vi "Add Procedure.vi"(7 "Overwrite Existing?":bool=TRUE, 8 "error in (no error)":errorcluster, 9 "Settings":cluster{"Name":string}, 10 "Base Node Path":string, 11 "SysDef Ref":T1) -> (0 "error out":errorcluster, 2 "New Node Path":string, 3 "SysDef Ref Out":T1)   [LabVIEW 2019, in "Simple SysDef API.lvlib"]
uses:
  <userlib>/SimpleSysDef/Simple SysDef API.lvlib
  <userlib>/SimpleSysDef/_SubVIs/System Definition Reference.ctl
  NationalInstruments.VeriStand.SystemDefinitionAPI
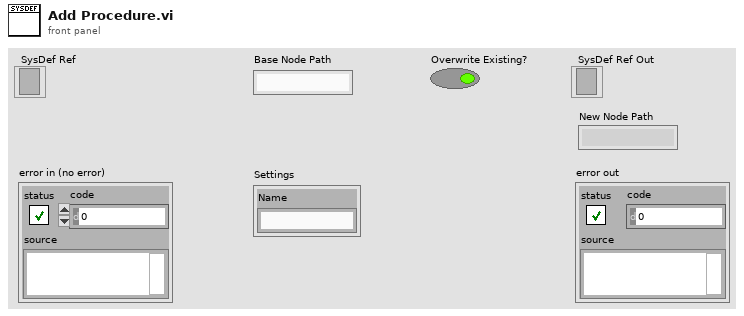
[diagram p1: front panel]
types:
  T1 = typedef "Simple SysDef API.lvlib/System Definition Reference.ctl" = refnum<k24>
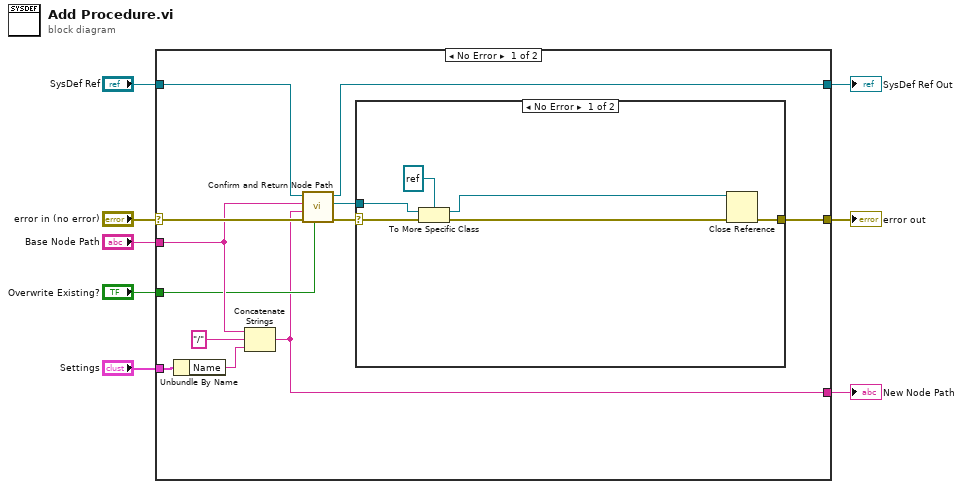
[diagram p0: block diagram]
diagram:
  n1 = case shown="No Error" "error in (no error)" {
    selector: "error in (no error)" -> [w20 w29]
    tunnel: [w14 w29] -> w7
    tunnel: "SysDef Ref" -> [w19 w28]
    tunnel: [w18 w28] -> w5
    tunnel: "Base Node Path" -> [w11 _]
    tunnel: "Overwrite Existing?" -> [w10 _]
    tunnel: "Settings" -> [w17 _]
    tunnel: [w9 _] -> w1
    frame No Error {
      n2 = Unbundle By Name(w17) -> ("Name"=w15:string)
      n3 = Concatenate Strings(w11, "/" ("string"), w15) -> (w9:string)
      n4 = call <userlib>:"Confirm and Return Node Path.vi"("Overwrite Existing?"=w10, "error in (no error)"=w20, "New Node Path"=w9, "Base Node Path"=w11, "SysDef Ref"=w19) -> ("error out"=w12:errorcluster, "Node Ref"=w13:refnum<k24>, "SysDef Ref Out"=w18:T1)  [unwired: 4 in]
      n5 = case shown="No Error" w12 {
        selector: w12 -> [w25 w27]
        tunnel: [w23 w27] -> w14
        tunnel: w13 -> [w26 _]
        frame No Error {
          n6 = To More Specific Class(target class=refnum<k24> refnum ("Node Ref"), reference=w26, error in=w25) -> (specific class reference=w22:refnum<k24>, error out=w24:errorcluster)
          n7 = Close Reference(reference=w22, error in (no error)=w24) -> (error out=w23:errorcluster)
        }
        frame Error {
        }
      }
    }
    frame Error {
    }
  }
  "SysDef Ref Out" <- w5
  "error out" <- w7
  "New Node Path" <- w1
